vi "Configure Source (Range).vi"(0 "VISA resource name":refnum<visa-resource-name>, 1 "Current Range (1E-7 A)":dbl=1e-07, 2 "Voltage Range (0.2 V)":dbl=0.2, 5 "Source Measure Unit Channel (0: Channel A)":i32(ring) items=["Channel A", "Channel B"], 7 "Range Type (1: Voltage)":i32(ring)=1 items=["Current", "Voltage"], 9 "Auto Range (T: Enable)":bool=TRUE, 11 "error in (no error)":errorcluster, 12 "Minimum Current  Range (1E-7 A)":dbl=1e-07, 13 "Minimum Voltage Range (0.2 V)":dbl=0.2) -> (4 "VISA resource name out":refnum<visa-resource-name>, 15 "error out":errorcluster)   [LabVIEW 2017, in "Keithley 2600 Series.lvlib"]
doc: "Configures the source range."
uses:
  <instrlib>/Keithley 2600 Series/Keithley 2600 Series.lvlib
panel:
  # "Auto Range Off"
  # "Auto Range On"
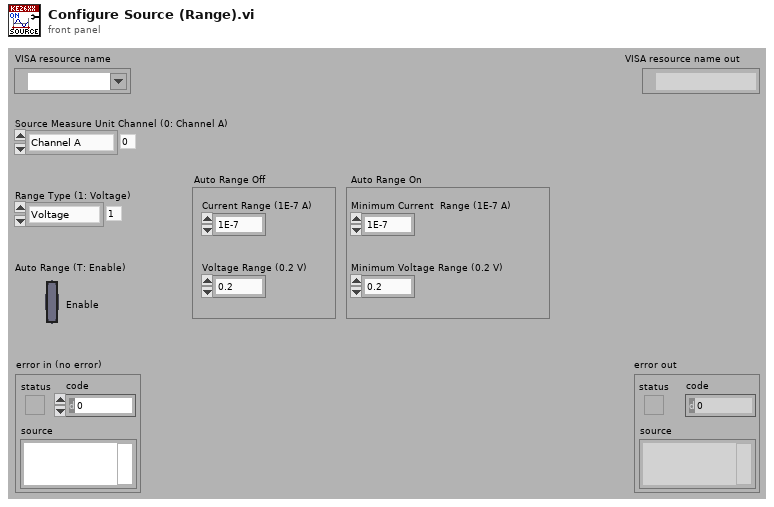
[diagram p1: front panel]
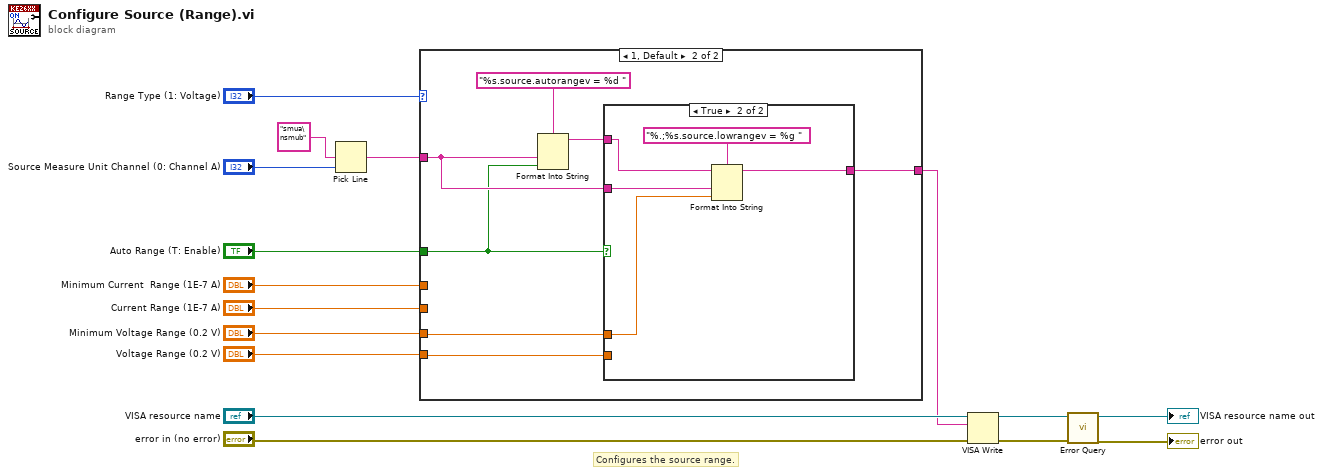
[diagram p0: block diagram]
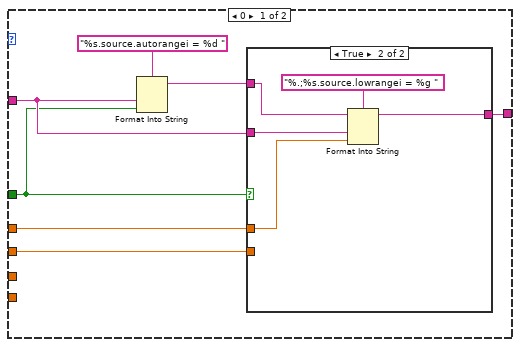
[diagram p2: hidden frame]
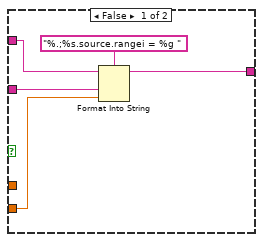
[diagram p3: hidden frame]
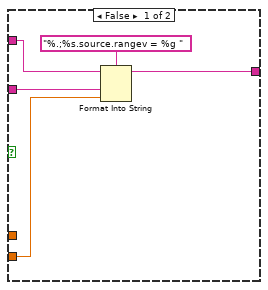
[diagram p4: hidden frame]
diagram:
  # "Configures the source range."
  n1 = Pick Line(multi-line string="smua\nsmub", line index="Source Measure Unit Channel (0: Channel A)") -> (output string=w8:string)  [unwired: 1 in]
  n2 = case shown="1, Default" "Range Type (1: Voltage)" {
    tunnel: w8 -> [w21 w38]
    tunnel: "Auto Range (T: Enable)" -> [w17 w34]
    tunnel: "Minimum Current  Range (1E-7 A)" -> [w20 _]
    tunnel: "Current Range (1E-7 A)" -> [w19 _]
    tunnel: [w18 w37] -> w1
    tunnel: "Minimum Voltage Range (0.2 V)" -> [_ w36]
    tunnel: "Voltage Range (0.2 V)" -> [_ w35]
    frame 0 {
      n3 = Format Into String(format string="%s.source.autorangei = %d ", w21, w17) -> (resulting string=w22:string)  [unwired: 2 in, 1 out]
      n4 = case shown="True" w17 {
        tunnel: w22 -> [w27 w32]
        tunnel: w21 -> [w25 w31]
        tunnel: w20 -> [_ w30]
        tunnel: w19 -> [w24 _]
        tunnel: [w26 w29] -> w18
        frame False {
          n5 = Format Into String(format string="%.;%s.source.rangei = %g ", initial string=w27, w25, w24) -> (resulting string=w26:string)  [unwired: 1 in, 1 out]
        }
        frame True {
          n6 = Format Into String(format string="%.;%s.source.lowrangei = %g ", initial string=w32, w31, w30) -> (resulting string=w29:string)  [unwired: 1 in, 1 out]
        }
      }
    }
    frame 1, Default {
      n7 = Format Into String(format string="%s.source.autorangev = %d ", w38, w34) -> (resulting string=w39:string)  [unwired: 2 in, 1 out]
      n8 = case shown="True" w34 {
        tunnel: w39 -> [w43 w46]
        tunnel: w38 -> [w42 w48]
        tunnel: [w41 w49] -> w37
        tunnel: w36 -> [_ w47]
        tunnel: w35 -> [w44 _]
        frame False {
          n9 = Format Into String(format string="%.;%s.source.rangev = %g ", initial string=w43, w42, w44) -> (resulting string=w41:string)  [unwired: 1 in, 1 out]
        }
        frame True {
          n10 = Format Into String(format string="%.;%s.source.lowrangev = %g ", initial string=w46, w48, w47) -> (resulting string=w49:string)  [unwired: 1 in, 1 out]
        }
      }
    }
  }
  n11 = VISA Write(VISA resource name="VISA resource name", write buffer=w1, error in (no error)="error in (no error)") -> (VISA resource name out=w14:refnum<visa-resource-name>, error out=w13:errorcluster)  [unwired: 1 out]
  n12 = call <instrlib>:"Error Query.vi"("error in (no error)"=w13, "VISA resource name"=w14) -> ("error out"=→"error out":errorcluster, "VISA resource name out"=→"VISA resource name out":refnum<visa-resource-name>)  [unwired: 6 in, 2 out]
